vi "RelativeLeadScrew (SubVI).vi"(8 "error in (no error)":errorcluster, 10 "Distance (cm)":dbl, 11 "miniOut in":T1) -> (0 "error out":errorcluster, 1 "LimitSW":bool, 2 "ENC Counter (deg/s)":dbl, 3 "miniOut out":T1)   [LabVIEW 2019]
uses:
  <vilib>/ReMiSYS/ReMiSYS_myRIO-mini/SubVI/SYS/miniRef.ctl
  <vilib>/Platform/TimedLoop/XDataNode/timing_clust.ctl
  <vilib>/Platform/TimedLoop/XDataNode/nitl_modes.ctl
  <vilib>/Platform/TimedLoop/XDataNode/wakeup.ctl
  <vilib>/platform/TimedLoop/XDataNode/XDataNode.xnode
  <vilib>/Platform/TimedLoop/XDataNode/XDNodeRunTimeDep.lvlib
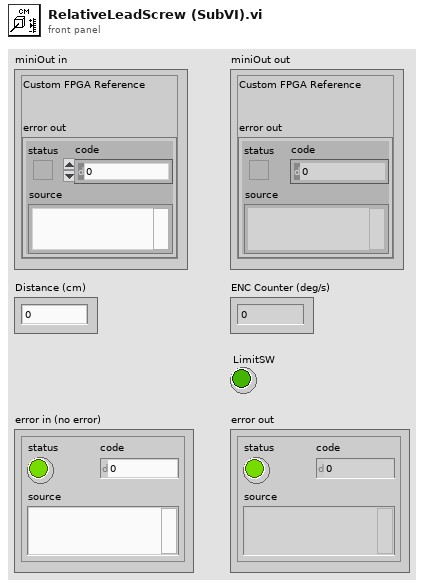
[diagram p1: front panel]
types:
  T1 = typedef "miniRef.ctl" = cluster{"Custom FPGA Reference":refnum<k20>, "error out":errorcluster}
  T2 = typedef "XDNodeRunTimeDep.lvlib/timing_clust.ctl" = cluster{"Expected End [f-1]":u64, "Actual End [f-1]":u64, "Finished Late? [f-1]":bool, "Expected End [i-1]":u64, "Actual End [i-1]":u64, "Finished Late? [i-1]":bool, "Expected Start [i]":u64, "Actual Start [i]":u64, "Expected Start [f]":u64, "Actual Start [f]":u64, "Source Name":string, "Structure Name":string, "Period":i64, "Deadline":i64, "Offset":i64, "Start":i64, "Priority":i32, "Timeout":i32, "Mode":T3, "Wakeup Reason":T4, "Error":errorcluster, "Source Type":string, "Secondary Source Type":string, "Global End Time":u64, "Global Start Time":u64, "Frame Duration":u64, "Iteration Duration":u64, "Assigned CPU":i32, "I/O Scan Engine Mode":u32}
  T3 = typedef "XDNodeRunTimeDep.lvlib/nitl_modes.ctl" = enum32{"No Change", "Process missed periods, maintain original phase", "Discard missed periods, maintain original phase", "Process missed periods, ignore original phase", "Discard missed periods, ignore original phase"}
  T4 = typedef "XDNodeRunTimeDep.lvlib/wakeup.ctl" = enum32{"Normal", "Aborted", "Asynchronous wakeup", "Timing source error", "Timed loop error", "Timeout"}
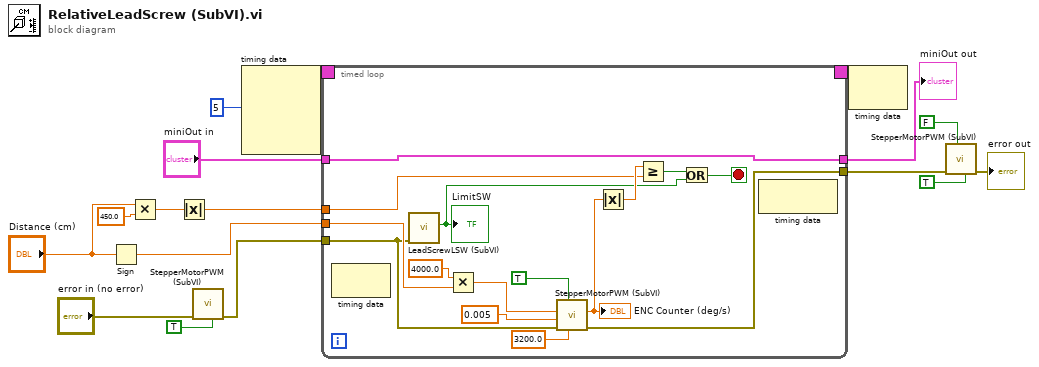
[diagram p0: block diagram]
diagram:
  n1 = Sign(1:"Distance (cm)") -> (0:w15:dbl)
  n2 = Multiply(x="Distance (cm)", y=450.0) -> (x*y=w12:dbl)
  n3 = Absolute Value(x=w12) -> (abs(x)=w13:dbl)
  n4 = call "StepperMotorPWM (SubVI).vi"("Reset"=TRUE, "error in (no error)"="error in (no error)") -> ("error out (no error)"=w3:errorcluster)  [unwired: 8 in, 1 out]
  n5 = node-c288(i64 5 ("Period")) -> (w17:T2)  [unwired: 3 in]
  n6 = timed-loop {
    timing: w17 -> [_]
    timing-out: [_] -> w16
    tunnel: [w32] -> w6
    tunnel: w3 -> [w21]
    tunnel: [w26] -> w8
    tunnel: "miniOut in" -> [w26]
    tunnel: w13 -> [w24]
    tunnel: w15 -> [w23]
    stop <- w28 stop-if-true
    n7 = node-c288() -> ()  [unwired: 1 in, 1 out]
    n8 = call "LeadScrewLSW (SubVI).vi"("error in (no error)"=w21) -> ("LeadScrewLimitSW"=w19:bool)  [unwired: 9 in, 1 out]
    "LimitSW" <- w19
    n9 = Multiply(x=4000.0 ("Speed (deg/s) [L,R]"), y=w23) -> (x*y=w22:dbl)
    n10 = call "StepperMotorPWM (SubVI).vi"("steps/rev"=3200.0, "EN"=TRUE, "error in (no error)"=w21, "LoopTime"=0.005, "Speed (deg/s) [L,R]"=w22) -> ("error out (no error)"=w32:errorcluster, "DegreeCounter"=w30:dbl)  [unwired: 5 in]
    "ENC Counter (deg/s)" <- w30
    n11 = Absolute Value(x=w30) -> (abs(x)=w25:dbl)
    n12 = Greater Or Equal?(x=w25, y=w24) -> (x >= y?=w29:bool)
    n13 = Or(x=w29, y=w19) -> (x .or. y?=w28:bool)
    n14 = node-c288() -> ()  [unwired: 1 in, 1 out]
  }
  "miniOut out" <- w8
  n15 = node-c288(w16) -> ()  [unwired: 1 out]
  n16 = call "StepperMotorPWM (SubVI).vi"("Reset"=TRUE, "EN"=FALSE ("EN [L,R]"), "error in (no error)"=w6) -> ("error out (no error)"=→"error out":errorcluster)  [unwired: 7 in, 1 out]
